vi "Volt Reader Trigger6.vi"() -> ()   [LabVIEW 2014]
uses:
  <vilib>/Utility/error.llb/DialogType.ctl
  <vilib>/_DAQmxBase/Internals/DAQmxBase Create Channel (AI-Voltage-Basic).vi
  <vilib>/_DAQmxBase/Internals/DAQmxBase Timing (Sample Clock).vi
  <vilib>/_DAQmxBase/Internals/DAQmxBase Read (Analog 2D DBL NChan NSamp).vi
panel:
  in  "Continue Graphing":bool
  in  "Knob amplifier":dbl
  in  "Enable Center":bool
  in  "Center Button":bool
  in  "Knob":dbl(knob) scale=0.0..1.0
  out "Waveform Graph":waveform(dbl)(graph)
  in  "Buffer (ms)":dbl
  out "Threshold":dbl
  in  "units":i32(ring)=10348 items=["Volts"=10348, "From Custom Scale"=10065]
  in  "stop":bool
  in  "physical channels":tag
  in  "maximum value":dbl=5.0 format="%0.2f"
  in  "minimum value":dbl=-5.0 format="%0.2f"
  in  "rate":i32=1000 caption="Sample Rate"
  # "The inputs above MUST BE\nPreset before running"
  # "NOTE: Just change the Y axis value"
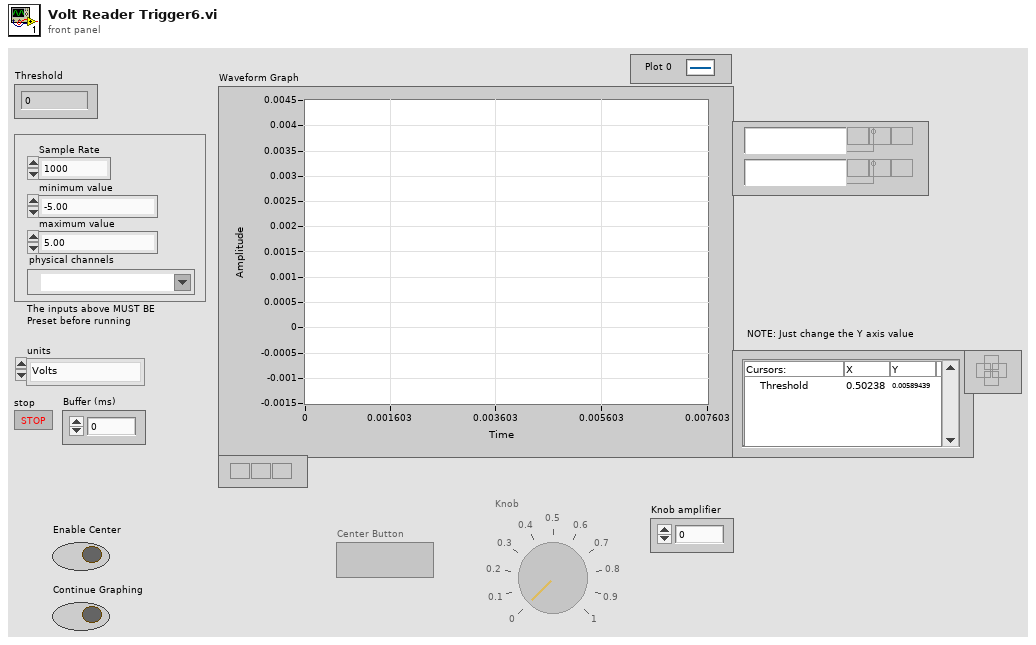
[diagram p1: front panel]
types:
  T1 = enum8{"Enabled", "Disabled", "Disabled and Grayed Out"}
  T2 = typedef "DialogType.ctl" = u16
  T3 = typedef "LVCursorListTypeDef.ctl" = cluster{"Name":string, "Color":u32, "Style":u8, "Point Style":u8, "Name Visible":bool, "Allow Drag":bool, "Cursor Mode":u32, "Plot":i32, "Index":i32, "Position":cluster{"X":dbl, "Y":dbl}, "X Scale":u32, "Y Scale":u32, "Watch Plots":i32[], "Watch All Plots":bool, "Plot Area":i32, "Label Offset":cluster{"X":dbl, "Y":dbl}}[]
  T4 = cluster{"Name":string, "Color":u32, "Style":u8, "Point Style":u8, "Name Visible":bool, "Allow Drag":bool, "Cursor Mode":u32, "Plot":i32, "Index":i32, "Position":cluster{"X":dbl, "Y":dbl}, "X Scale":u32, "Y Scale":u32, "Watch Plots":i32[], "Watch All Plots":bool, "Plot Area":i32, "Label Offset":cluster{"X":dbl, "Y":dbl}}
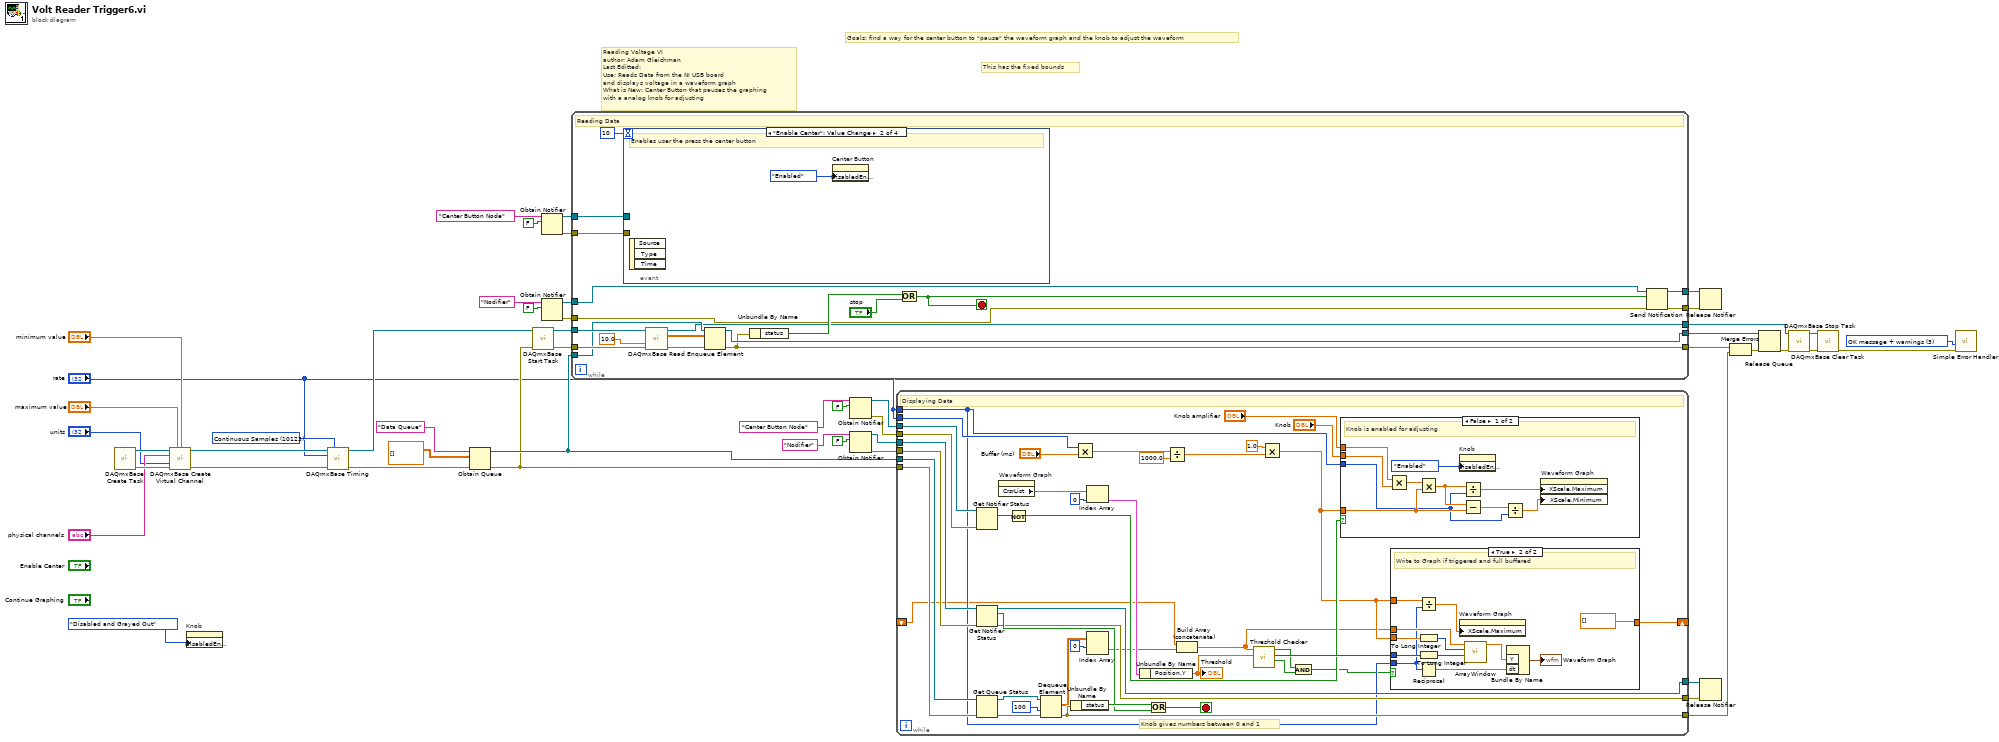
[diagram p0: block diagram]
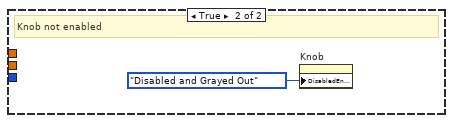
[diagram p2: hidden frame]
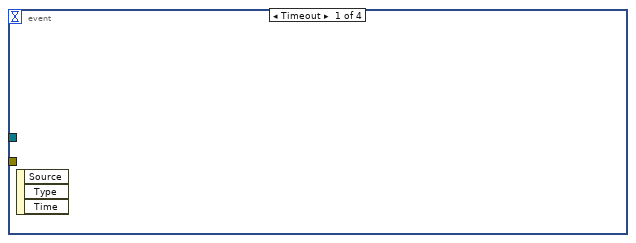
[diagram p4: hidden frame]
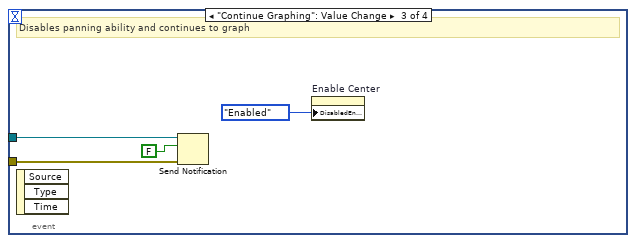
[diagram p5: hidden frame]
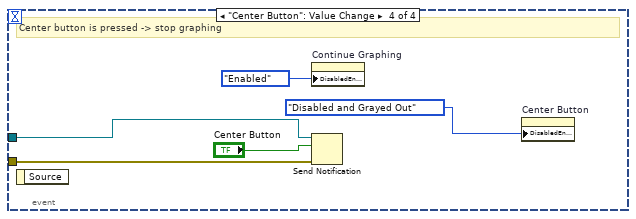
[diagram p6: hidden frame]
diagram:
  w26 = 10123 items=["Finite Samples"=10178, "Continuous Samples"=10123, "Hardware Timed Single Point"=12522] ("sample mode")
  w28 = T2 3 items=["no dialog", "OK message", "continue or stop message", "OK message + warnings", "continue/stop + warnings"] ("type of dialog (OK msg:1)")
  # "Goals: find a way for the center button to \"pause\" the waveform graph and the knob to adjust the waveform"
  # "This has the fixed bounds"
  # "Reading Voltage VI\nauthor: Adam Gleichman\nLast Editted: \nUse: Reads Data from the NI USB board\nand displays voltage in a waveform graph\nWhat is New: Center Button that pauses the graphing\nwith a analog knob for adjusting"
  n1 = call <vilib>:"DAQmxBase Create Task.vi"() -> ("task out"=w48:refnum<k21>, "error out"=w47:errorcluster)  [unwired: 5 in, 9 out]
  n2 = call-poly <vilib>:"DAQmxBase Create Virtual Channel.vi"("task in"=w48, "maximum value"="maximum value", "minimum value"="minimum value", "physical channels"="physical channels", "units"="units", "error in"=w47) -> ("task out"=w45:refnum<k21>, "error out"=w46:errorcluster)  [unwired: 3 in, 5 out]
  n3 = property on="Knob" class="Knob (strict)"("DisabledEnum"=T1."Disabled and Grayed Out" ("Disabled")) -> ()  [unwired: 2 in, 2 out]
  n4 = call-poly <vilib>:"DAQmxBase Timing.vi"("task/channels in"=w45, "sample mode"=w26, "rate"="rate", "error in"=w46) -> ("task out"=w14:refnum<k21>, "error out"=w13:errorcluster)  [unwired: 3 in, 7 out]
  n5 = Obtain Queue(name (unnamed)="Data Queue", element data type=dbl[][] [] ("data"), error in (no error)=w13) -> (queue out=w35:refnum<queue>, error out=w34:errorcluster)  [unwired: 2 in, 1 out]
  n6 = call <vilib>:"DAQmxBase Start Task.vi"("task/channels in"=w14, "error in"=w34) -> ("task out"=w43:refnum<k21>, "error out"=w44:errorcluster)  [unwired: 12 out]
  n7 = Obtain Notifier(name (unnamed)="Center Button Node", notification data type=FALSE) -> (notifier out=w11:refnum<notifier>, error out=w10:errorcluster)  [unwired: 2 in, 1 out]
  n8 = Obtain Notifier(name (unnamed)="Nodifier", notification data type=FALSE) -> (notifier out=w22:refnum<notifier>, error out=w21:errorcluster)  [unwired: 2 in, 1 out]
  n9 = while "Data Reading Loop" {
    tunnel: w44 -> [w67]
    tunnel: w43 -> [w68]
    tunnel: w35 -> [w65]
    tunnel: [w62] -> w38
    tunnel: [w60] -> w37
    tunnel: [w58] -> w25
    tunnel: w22 -> [w56]
    tunnel: w21 -> [w55]
    tunnel: w11 -> [w54]
    tunnel: w10 -> [w53]
    tunnel: [w51] -> w3
    tunnel: [w50] -> w2
    stop <- w57 stop-if-true
    # "Reading Data"
    n10 = event shown="[1] \"Enable Center\": Value Change" {
      selector: _ -> [_ _ _ _]
      dyn-events: _ -> [_ _ _ _]
      timeout: 10 -> [_ _ _ _]
      tunnel: w54 -> [_ _ w72 w78]
      tunnel: w53 -> [_ _ w71 w77]
      event Timeout {
        n11 = event-data() -> ()  [unwired: 1 in, 3 out]
      }
      event "Enable Center": Value Change {
        # "Enables user the press the center button"
        n12 = event-data() -> ()  [unwired: 1 in, 3 out]
        n13 = property on="Center Button" class="Bool"("DisabledEnum"=T1."Enabled" ("Disabled")) -> ()  [unwired: 2 in, 2 out]
      }
      event "Continue Graphing": Value Change {
        # "Disables panning ability and continues to graph"
        n14 = event-data() -> ()  [unwired: 1 in, 3 out]
        n15 = Send Notification(notification=FALSE, notifier=w72, error in (no error)=w71) -> ()  [unwired: 2 out]
        n16 = property on="Enable Center" class="Bool (strict)"("DisabledEnum"=T1."Enabled" ("Disabled")) -> ()  [unwired: 2 in, 2 out]
      }
      event "Center Button": Value Change {
        # "Center button is pressed -> stop graphing"
        n17 = event-data() -> ()  [unwired: 1 in, 1 out]
        n18 = property on="Continue Graphing" class="Bool (strict)"("DisabledEnum"=T1."Enabled" ("Disabled")) -> ()  [unwired: 2 in, 2 out]
        n19 = Send Notification(notification="Center Button", notifier=w78, error in (no error)=w77) -> ()  [unwired: 2 out]
        n20 = property on="Center Button" class="Bool"("DisabledEnum"=T1."Disabled and Grayed Out" ("Disabled")) -> ()  [unwired: 2 in, 2 out]
      }
    }
    n21 = call-poly <vilib>:"DAQmxBase Read.vi"("task/channels in"=w68, "timeout"=10.0, "error in"=w67) -> ("task out"=w58:refnum<k21>, "data"=w63:dbl[][], "error out"=w66:errorcluster)  [unwired: 10 in]
    n22 = Enqueue Element(queue=w65, element=w63, error in (no error)=w66) -> (queue out=w62:refnum<queue>, error out=w60:errorcluster)  [unwired: 1 in, 1 out]
    n23 = Unbundle By Name(w60) -> ("status"=w59:bool)
    n24 = Or(x=w59, y="stop") -> (x .or. y?=w57:bool)
    n25 = Send Notification(notification=w57, notifier=w56, error in (no error)=w55) -> (notifier out=w51:refnum<notifier>, error out=w50:errorcluster)
  }
  n26 = Obtain Notifier(name (unnamed)="Center Button Node", notification data type=FALSE) -> (notifier out=w1:refnum<notifier>, error out=w5:errorcluster)  [unwired: 2 in, 1 out]
  n27 = Obtain Notifier(name (unnamed)="Nodifier", notification data type=FALSE) -> (notifier out=w19:refnum<notifier>, error out=w17:errorcluster)  [unwired: 2 in, 1 out]
  n28 = while {
    tunnel: w35 -> [w119]
    tunnel: w34 -> [w108]
    tunnel: [w117] -> w33
    tunnel: w19 -> [w114]
    tunnel: w17 -> [w113]
    tunnel: [w111] -> w15
    tunnel: [w110] -> w16
    tunnel: "rate" -> [w85]
    tunnel: "rate" -> [w97]
    tunnel: w1 -> [w87]
    tunnel: w5 -> [w91]
    shift-right: [w80] -> _
    shift-left: _ -> [w79]
    stop <- w115 stop-if-true
    # "Knob gives numbers between 0 and 1"
    # "Displaying Data"
    n29 = Get Notifier Status(notifier=w87, error in (no error)=w91) -> (current notification=w90:bool)  [unwired: 4 out]
    n30 = Get Notifier Status(notifier=w114, error in (no error)=w113) -> (notifier out=w111:refnum<notifier>, current notification=w112:bool, error out=w110:errorcluster)  [unwired: 2 out]
    n31 = Get Queue Status(queue=w119, error in (no error)=w108) -> (queue out=w109:refnum<queue>, error out=w107:errorcluster)  [unwired: 1 in, 6 out]
    n32 = property on="Waveform Graph" class="WFGraph (strict)"() -> ("CrsrList"=w102:T3)  [unwired: 2 in, 2 out]
    n33 = Not(x=w90) -> (.not. x?=w88:bool)
    n34 = Dequeue Element(queue=w109, timeout in ms (-1)=100, error in (no error)=w107) -> (element=w105:dbl[][], error out=w117:errorcluster)  [unwired: 2 out]
    n35 = Unbundle By Name(w117) -> ("status"=w116:bool)
    n36 = Multiply(x=w97, y="Buffer (ms)") -> (x*y=w99:dbl)
    n37 = Index Array(array=w102, index=0) -> (element=w101:T4)
    n38 = Index Array(array=w105, index (row)=0 ("index")) -> (element=w82:dbl[])  [unwired: 1 in]
    n39 = Unbundle By Name(w101) -> ("Position.Y"=w100:dbl)
    "Threshold" <- w100
    n40 = Or(x=w116, y=w112) -> (x .or. y?=w115:bool)
    n41 = Divide(x=w99, y=1000.0) -> (x/y=w96:dbl)
    n42 = Build Array (concatenate)(w79, w82) -> (w81:dbl[])
    n43 = call "Threshold Checker.vi"("Threshold"=w100, "Data"=w81) -> ("buffer filled?"=w92:bool, "Index of Value = to or exceeding threshold"=w104:i32, "Did we pass the threshold?"=w93:bool)  [unwired: 7 in]
    n44 = Multiply(x=1.0, y=w96) -> (x*y=w86:dbl)
    n45 = And(x=w93, y=w92) -> (x .and. y?=w83:bool)
    n46 = case shown="False" w88 {
      tunnel: "Knob" -> [w127 _]
      tunnel: "Knob amplifier" -> [w128 _]
      tunnel: w86 -> [w125 _]
      tunnel: w85 -> [w120 _]
      frame False {
        # "Knob is enabled for adjusting"
        n47 = Multiply(x=w128, y=w127) -> (x*y=w126:dbl)
        n48 = Multiply(x=w126, y=w125) -> (x*y=w123:dbl)
        n49 = property on="Knob" class="Knob (strict)"("DisabledEnum"=T1."Enabled" ("Disabled")) -> ()  [unwired: 2 in, 2 out]
        n50 = Divide(x=w123, y=w120) -> (x/y=w121:dbl)
        n51 = Subtract(x=w123, y=w125) -> (x-y=w124:dbl)
        n52 = Divide(x=w124, y=w120) -> (x/y=w122:dbl)
        n53 = property on="Waveform Graph" class="WFGraph (strict)"("XScale.Maximum"=w121, "XScale.Minimum"=w122) -> ()  [unwired: 2 in, 2 out]
      }
      frame True {
        # "Knob not enabled"
        n54 = property on="Knob" class="Knob (strict)"("DisabledEnum"=T1."Disabled and Grayed Out" ("Disabled")) -> ()  [unwired: 2 in, 2 out]
      }
    }
    n55 = case shown="True" w83 {
      tunnel: w86 -> [_ w140]
      tunnel: w104 -> [_ w139]
      tunnel: w85 -> [_ w134]
      tunnel: w81 -> [w131 w136]
      tunnel: w86 -> [_ w135]
      tunnel: [w131 dbl[] []] -> w80
      frame False {
        # "Write nothing on the graph"
      }
      frame True {
        # "Write to Graph if triggered and full buffered"
        n56 = Divide(x=w135, y=w134) -> (x/y=w133:dbl)
        n57 = To Long Integer(number=w140) -> (32bit integer=w137:i32)
        n58 = To Long Integer(number=w139) -> (32bit integer=w138:i32)
        n59 = Reciprocal(x=w134) -> (1/x=w143:dbl)
        n60 = property on="Waveform Graph" class="WFGraph (strict)"("XScale.Maximum"=w133) -> ()  [unwired: 2 in, 2 out]
        n61 = call "ArrayWindow.VI"("Index"=w138, "Total amount of Pts"=w137, "Input Y-values"=w136) -> ("Output Array"=w141:dbl[])  [unwired: 8 in]
        n62 = Bundle By Name("Y"=w141, "dt"=w143) -> (→"Waveform Graph":waveform(dbl))  [unwired: 1 in]
      }
    }
  }
  n63 = Release Notifier(notifier=w3, error in (no error)=w2) -> ()  [unwired: 1 in, 3 out]
  n64 = Release Notifier(notifier=w15, error in (no error)=w16) -> ()  [unwired: 1 in, 3 out]
  n65 = Merge Errors(w37, w33) -> (w36:errorcluster)
  n66 = Release Queue(queue=w38, error in (no error)=w36) -> (error out=w32:errorcluster)  [unwired: 1 in, 2 out]
  n67 = call <vilib>:"DAQmxBase Stop Task.vi"("task/channels in"=w25, "error in"=w32) -> ("task out"=w31:refnum<k21>, "error out"=w30:errorcluster)  [unwired: 12 in]
  n68 = call <vilib>:"DAQmxBase Clear Task.vi"("task in"=w31, "error in"=w30) -> ("error out"=w29:errorcluster)  [unwired: 13 in]
  n69 = call <vilib>:"Simple Error Handler.vi"("type of dialog (OK msg:1)"=w28, "error in (no error)"=w29) -> ()  [unwired: 3 in, 5 out]
